vi "SP_Action_Taken_Report.vi"() -> ()   [LabVIEW 2017]
uses:
  <vilib>/addons/database/Connection.llb/DB Tools Open Connec (Path).vi
  Globle/Login Data.vi
  <vilib>/addons/database/NI_Database_API.lvlib
panel:
  in  "Cancel Button - Archive":bool
  out "Role Id":string
  out "stackholder":string
  in  "Download 2":bool
  in  "Get Rport":bool
  out "index of element":i32
  out "Table 2":string[][](array[string])
  in  "Station":string(combo)
  out "error out":errorcluster
  in  "error in (no error)":errorcluster
  out "Table":string[][](table)
  out "Run-Time Status":cluster{"Array 2":timestamp[], dbl[]}(graph)
  in  "Shift":string(combo)
  in  "To Date":timestamp format="%<%Y-%m-%d>T"
  in  "From Date":timestamp format="%<%Y-%m-%d>T"
  in  "Stakeholder":string(combo)
  # "Breakdown & Action Taken Report"
  # "Powered By - Infinity Automation Systems Pvt. Ltd."
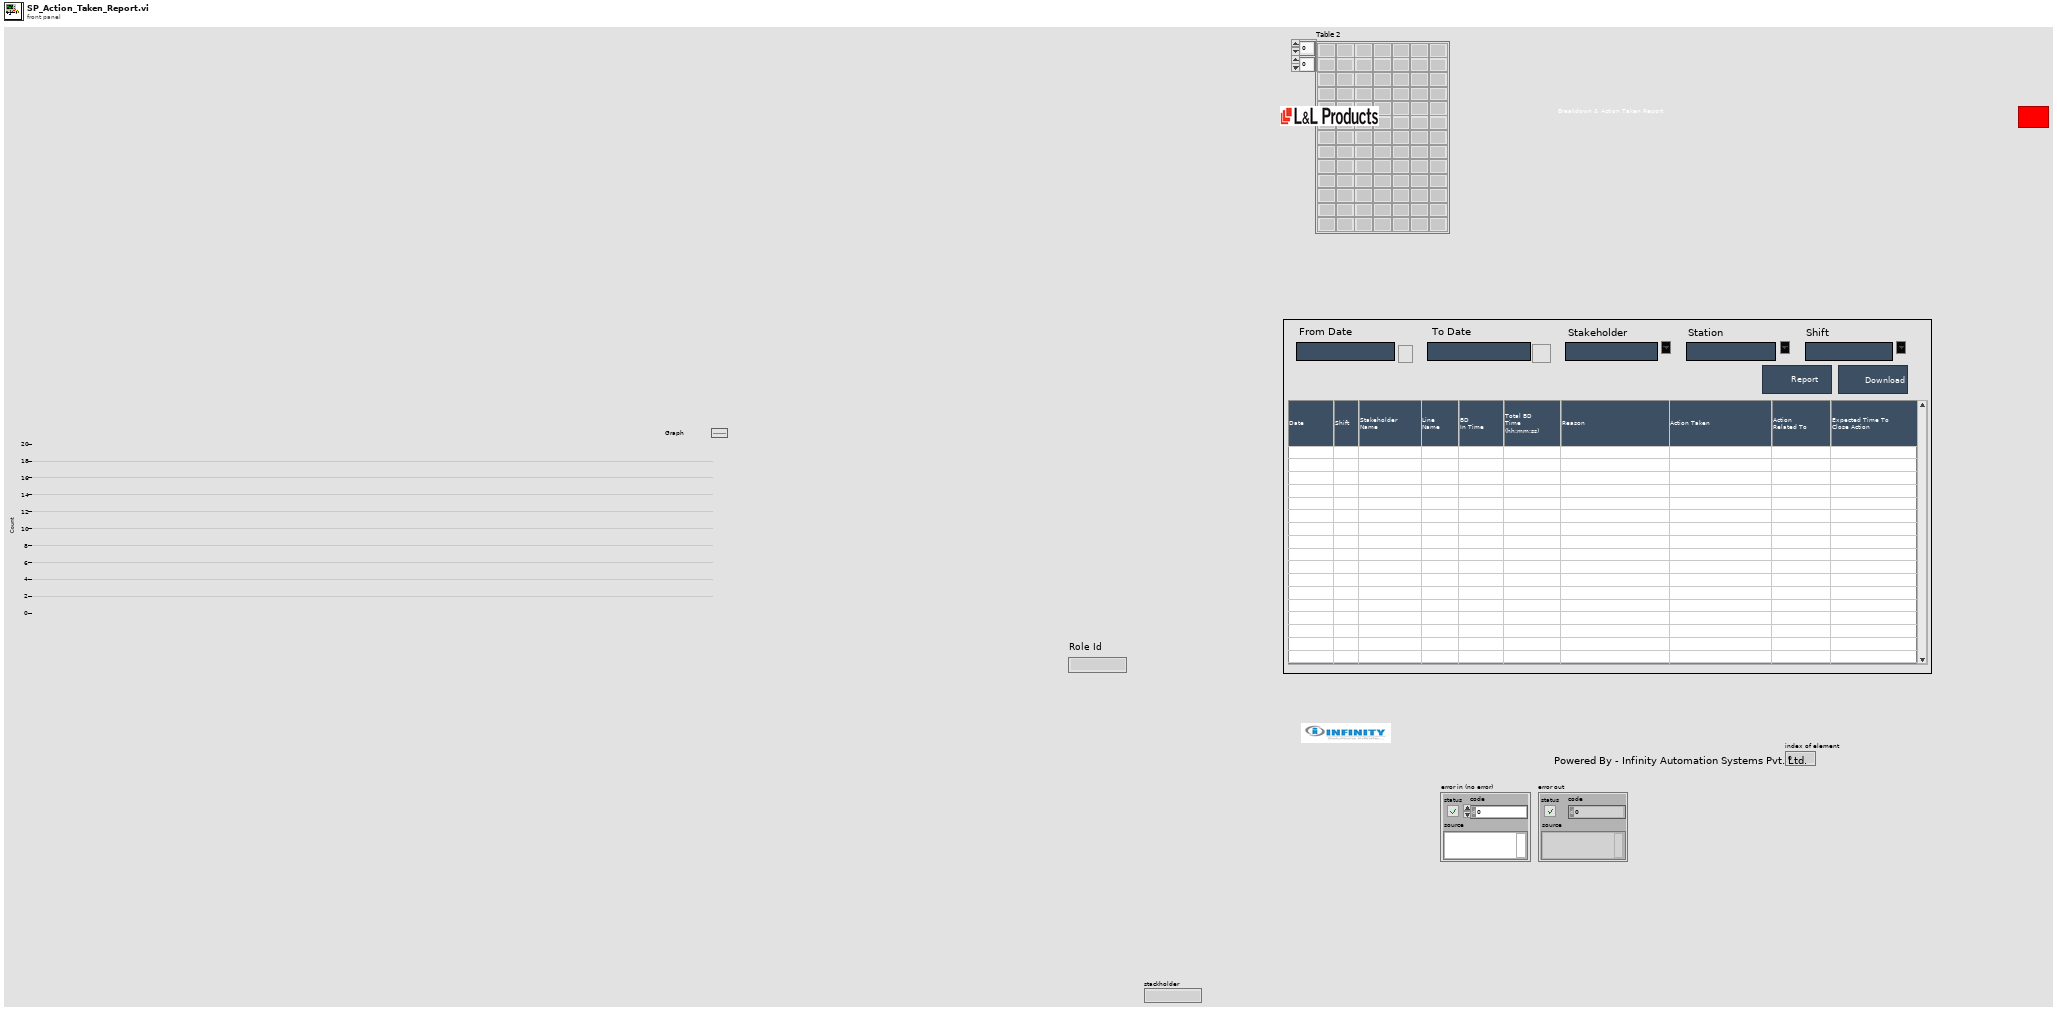
[diagram p1: front panel]
types:
  T1 = typedef "NI_Database_API.lvlib/Conn ObjectReference.ctl" = refnum<k1>
  T2 = enum32{"invalid app kind", "Development System", "Run Time System", "Student Edition", "Embedded LabVIEW", "Evaluation", "Custom"}
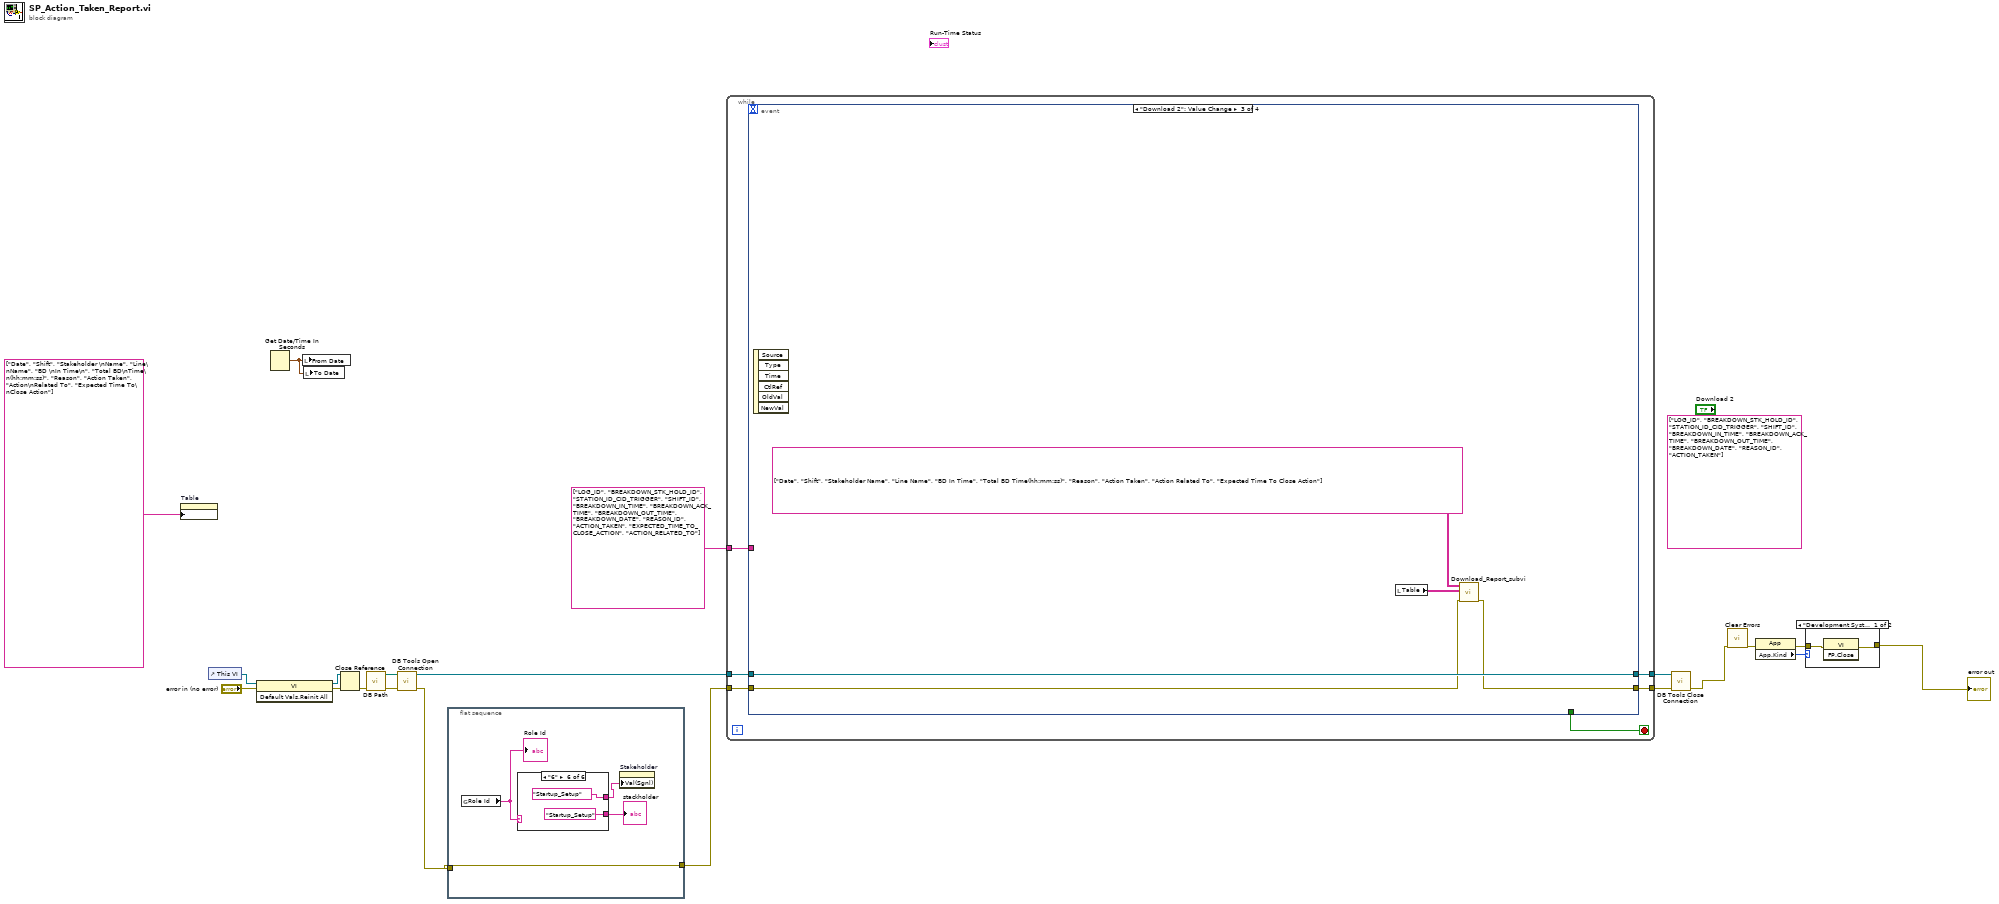
[diagram p0: block diagram]
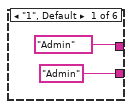
[diagram p2: hidden frame]
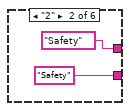
[diagram p3: hidden frame]
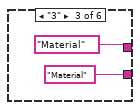
[diagram p4: hidden frame]
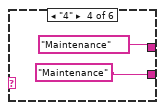
[diagram p5: hidden frame]
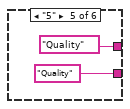
[diagram p6: hidden frame]
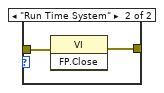
[diagram p7: hidden frame]
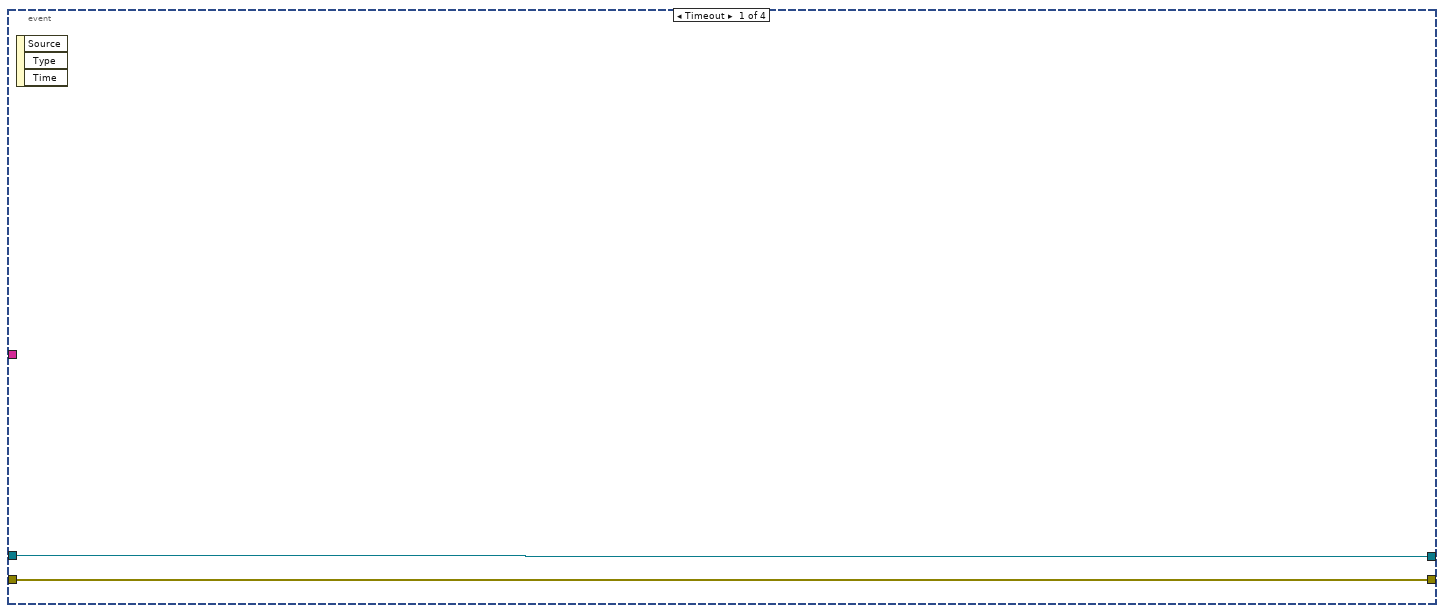
[diagram p8: hidden frame]
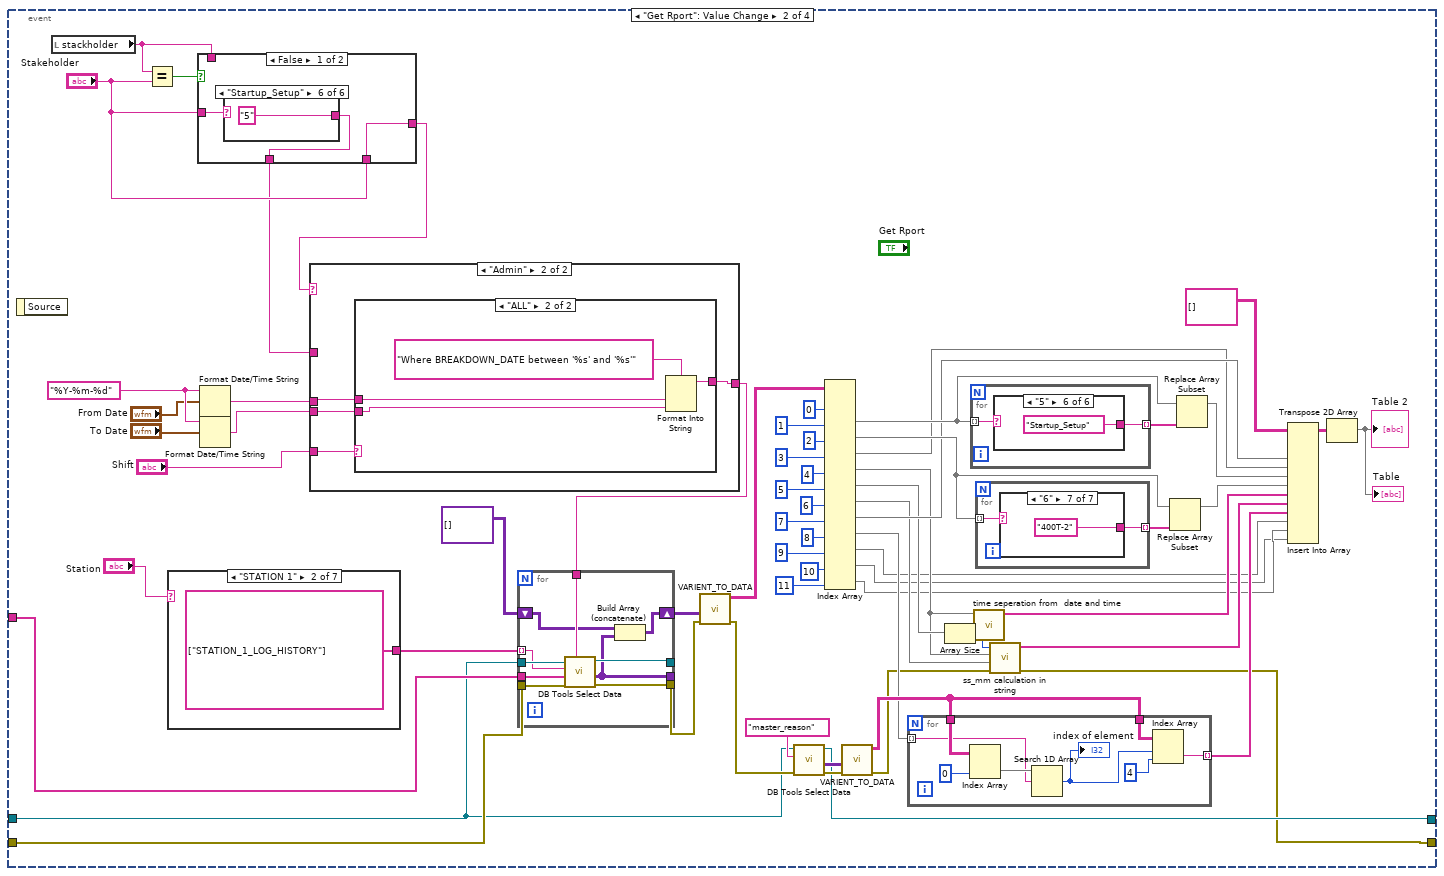
[diagram p9: hidden frame]
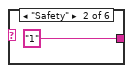
[diagram p11: hidden frame]
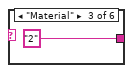
[diagram p12: hidden frame]
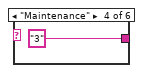
[diagram p13: hidden frame]
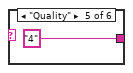
[diagram p14: hidden frame]
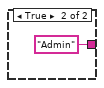
[diagram p15: hidden frame]
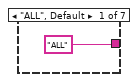
[diagram p16: hidden frame]
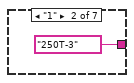
[diagram p17: hidden frame]
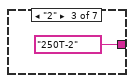
[diagram p18: hidden frame]
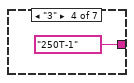
[diagram p19: hidden frame]
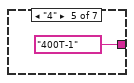
[diagram p20: hidden frame]
diagram:
  (unwired) string[] ["LOG_ID", "BREAKDOWN_STK_HOLD_ID", "STATION_ID_CID_TRIGGER", "SHIFT_ID", "BREAKDOWN_IN_TIME", "BREAKDOWN_ACK_TIME", "BREAKDOWN_OUT_TIME", "BREAKDOWN_DATE", "REASON_ID", "ACTION_TAKEN"]
  n1 = property on="Table" class="Tbl (strict)"("Column Headers[]"=string[] ["Date", "Shift", "Stakeholder \nName", "Line\nName", "BD \nIn Time\n", "Total BD\nTime\n(hh:mm:ss)", "Reason", "Action Taken", "Action\nRelated To", "Expected Time To\nClose Action"] ("Column Header Strings[]")) -> ()  [unwired: 2 in, 2 out]
  n2 = control-ref of="This VI"() -> (w20:refnum<vi>)
  n3 = invoke class="VI" method="Default Vals.Reinit All"(reference=w20, error in="error in (no error)") -> (reference out=w18:refnum<vi>, error out=w19:errorcluster)  [unwired: 1 in, 1 out]
  n4 = Get Date/Time In Seconds() -> (seconds since 1Jan1904=w9:timestamp)
  n5 = local write "From Date"(w9) -> ()
  n6 = local write "To Date"(w9) -> ()
  n7 = Close Reference(reference=w18, error in (no error)=w19) -> (error out=w17:errorcluster)
  n8 = call "DB Path.vi"("error in"=w17) -> ("error out"=w16:errorcluster, "DB Path"=w15:path)  [unwired: 9 in]
  n9 = call-poly <vilib>:"DB Tools Open Connection.vi"("error in (no error)"=w16, "connection information"=w15) -> ("error out"=w2:errorcluster, "connection reference"=w13:T1)  [unwired: 6 in]
  n10 = flat-sequence {
    tunnel: [w24] -> w1
    tunnel: w2 -> [w24]
    frame #0 {
      n11 = global read "Login Data.vi" "Role Id"() -> (w21:string)
      "Role Id" <- w21
      n12 = case shown="\"6\"" w21 {
        tunnel: ["Admin" ("string") "Safety" "Material" "Maintenance" "Quality" "Startup_Setup"] -> w22
        tunnel: ["Admin" ("Stakeholder") "Safety" ("Stakeholder") "Material" ("Stakeholder") "Maintenance" ("Stakeholder") "Quality" ("Stakeholder") "Startup_Setup" ("Stakeholder")] -> w23
        frame "1", Default {
        }
        frame "2" {
        }
        frame "3" {
        }
        frame "4" {
        }
        frame "5" {
        }
        frame "6" {
        }
      }
      "stackholder" <- w22
      n13 = property on="Stakeholder" class="CmbBox"("Val(Sgnl)"=w23) -> ()  [unwired: 2 in, 2 out]
    }
  }
  n14 = while {
    tunnel: w1 -> [w42]
    tunnel: [w41] -> w11
    tunnel: [w40] -> w10
    tunnel: w13 -> [w39]
    tunnel: string[] ["LOG_ID", "BREAKDOWN_STK_HOLD_ID", "STATION_ID_CID_TRIGGER", "SHIFT_ID", "BREAKDOWN_IN_TIME", "BREAKDOWN_ACK_TIME", "BREAKDOWN_OUT_TIME", "BREAKDOWN_DATE", "REASON_ID", "ACTION_TAKEN", "EXPECTED_TIME_TO_CLOSE_ACTION", "ACTION_RELATED_TO"] -> [w38]
    stop <- w37 stop-if-true
    n15 = event shown="[2] \"Download 2\": Value Change" {
      selector: _ -> [_ _ _ _]
      dyn-events: _ -> [_ _ _ _]
      timeout: _ -> [_ _ _ _]
      tunnel: [w44 w57 w189 w195] -> w41
      tunnel: w42 -> [w44 w98 w190 w195]
      tunnel: [w43 w60 w192 w194] -> w40
      tunnel: w39 -> [w43 w61 w192 w194]
      tunnel: w38 -> [_ w96 _ _]
      tunnel: [_ _ _ "Cancel Button - Archive"] -> w37
      event Timeout {
        n16 = event-data() -> ()  [unwired: 1 in, 3 out]
      }
      event "Get Rport": Value Change {
        w107 = "%Y-%m-%d" ("time format string (%c)")
        n17 = event-data() -> ()  [unwired: 1 in, 1 out]
        n18 = local read "stackholder"() -> (w49:string)
        n19 = Equal?(x=w49, y="Stakeholder") -> (x = y?=w53:bool)
        n20 = case shown="\"STATION 1\"" "Station" {
          tunnel: [string[] ["STATION_1_LOG_HISTORY", "STATION_2_LOG_HISTORY", "STATION_3_LOG_HISTORY", "STATION_4_LOG_HISTORY", "STATION_5_LOG_HISTORY", "STATION_6_LOG_HISTORY"] string[] ["STATION_1_LOG_HISTORY"] string[] ["STATION_2_LOG_HISTORY"] string[] ["STATION_3_LOG_HISTORY"] string[] ["STATION_4_LOG_HISTORY"] string[] ["STATION_5_LOG_HISTORY"] string[] ["STATION_6_LOG_HISTORY"]] -> w97
          frame "ALL", Default {
          }
          frame "STATION 1" {
          }
          frame "STATION 2" {
          }
          frame "STATION 3" {
          }
          frame "STATION 4" {
          }
          frame "STATION 5" {
          }
          frame "STATION 6" {
          }
        }
        n21 = case shown="False" w53 {
          tunnel: [w109 "Admin" ("Stakeholder")] -> w51
          tunnel: "Stakeholder" -> [w110 _]
          tunnel: w49 -> [_ _]
          tunnel: "Stakeholder" -> [w109 _]
          tunnel: [w108 _] -> w50
          frame False {
            n22 = case shown="\"Startup_Setup\"" w110 {
              tunnel: [_ "1" "2" "3" "4" "5"] -> w108
              frame "Admin", Default {
              }
              frame "Safety" {
              }
              frame "Material" {
              }
              frame "Maintenance" {
              }
              frame "Quality" {
              }
              frame "Startup_Setup" {
              }
            }
          }
          frame True {
          }
        }
        n23 = Format Date/Time String(time format string (%c)=w107, seconds (now)="From Date") -> (date/time string=w103:string)  [unwired: 1 in]
        n24 = Format Date/Time String(time format string (%c)=w107, seconds (now)="To Date") -> (date/time string=w102:string)  [unwired: 1 in]
        n25 = case shown="\"Admin\"" w51 {
          tunnel: [w162 w178] -> w99
          tunnel: "Shift" -> [w163 w177]
          tunnel: w103 -> [w161 w176]
          tunnel: w102 -> [w160 w175]
          tunnel: w50 -> [w159 _]
          frame "False", Default {
            n26 = case shown="\"ALL\"" w163 {
              selector: w163 -> [w164 _]
              tunnel: [w168 w173] -> w162
              tunnel: w161 -> [w167 w172]
              tunnel: w160 -> [w166 w171]
              tunnel: w159 -> [w165 w170]
              frame "False", Default {
                n27 = Format Into String(format string="Where BREAKDOWN_DATE between '%s' and '%s' and BREAKDOWN_STK_HOLD_ID ='%s'  and SHIFT_ID='%s'  " ("condition"), w167, w166, w165, w164) -> (resulting string=w168:string)  [unwired: 2 in, 1 out]
              }
              frame "ALL" {
                n28 = Format Into String(format string="Where BREAKDOWN_DATE between '%s' and '%s' and BREAKDOWN_STK_HOLD_ID = '%s' " ("condition"), w172, w171, w170) -> (resulting string=w173:string)  [unwired: 2 in, 1 out]
              }
            }
          }
          frame "Admin" {
            n29 = case shown="\"ALL\"" w177 {
              selector: w177 -> [w179 _]
              tunnel: [w182 w186] -> w178
              tunnel: w176 -> [w181 w185]
              tunnel: w175 -> [w180 w184]
              frame "False", Default {
                n30 = Format Into String(format string="Where BREAKDOWN_DATE between '%s' and '%s' and SHIFT_ID='%s'  " ("condition"), w181, w180, w179) -> (resulting string=w182:string)  [unwired: 2 in, 1 out]
              }
              frame "ALL" {
                n31 = Format Into String(format string="Where BREAKDOWN_DATE between '%s' and '%s'" ("condition"), w185, w184) -> (resulting string=w186:string)  [unwired: 2 in, 1 out]
              }
            }
          }
        }
        n32 = for {
          tunnel: w97 -> [w149] mode=indexing
          tunnel: [w143] -> _
          tunnel: w96 -> [w145]
          tunnel: w99 -> [w146]
          tunnel: w98 -> [w148]
          tunnel: [w147] -> w81
          tunnel: w61 -> [w151]
          tunnel: [w150] -> _
          shift-right: [w142] -> w80
          shift-left: variant[][] [] ("data") -> [w144]
          n33 = call <vilib>:"DB Tools Select Data.vi"("condition"=w146, "error in (no error)"=w148, "columns"=w145, "table"=w149, "connection reference"=w151) -> ("error out"=w147:errorcluster, "data"=w143:variant[][], "connection reference out"=w150:T1)  [unwired: 1 in]
          n34 = Build Array (concatenate)(w144, w143) -> (w142:variant[][])
        }
        n35 = call "VARIENT_TO_DATA.vi"("data"=w80, "error in (no error)"=w81) -> ("Table"=w79:string[][], "error out"=w65:errorcluster)  [unwired: 7 in]
        n36 = call <vilib>:"DB Tools Select Data.vi"("error in (no error)"=w65, "table"="master_reason", "connection reference"=w61) -> ("error out"=w67:errorcluster, "data"=w66:variant[][], "connection reference out"=w60:T1)  [unwired: 3 in]
        n37 = Index Array(array=w79, index (col) #1=0 ("disabled index (col)"), index (col) #2=1 ("disabled index (col)"), index (col) #3=2 ("disabled index (col)"), index (col) #4=3 ("disabled index (col)"), index (col) #5=4 ("disabled index (col)"), index (col) #6=5 ("disabled index (col)"), index (col) #7=6 ("disabled index (col)"), index (col) #8=7 ("disabled index (col)"), index (col) #9=8 ("disabled index (col)"), index (col) #10=9 ("disabled index (col)"), index (col) #11=10 ("disabled index (col)"), index (col) #12=11 ("disabled index (col)")) -> (element #2=w92:string[], element #3=w90:string[], element #4=w77:string[], element #5=w70:string[], element #6=w71:string[], element #7=w73:string[], element #8=w78:string[], element #9=w63:string[], element #10=w54:string[], element #11=w45:string[], element #12=w46:string[])  [unwired: 12 in, 1 out]
        n38 = call "VARIENT_TO_DATA.vi"("data"=w66, "error in (no error)"=w67) -> ("Table"=w64:string[][], "error out"=w58:errorcluster)  [unwired: 7 in]
        n39 = for {
          tunnel: [w120] -> w62 mode=indexing
          tunnel: w64 -> [w119]
          tunnel: w64 -> [w118]
          tunnel: w63 -> [w117] mode=indexing
          n40 = Index Array(array=w119, index (col)=0 ("disabled index (col)")) -> (element=w123:string[])  [unwired: 1 in]
          n41 = Search 1D Array(1D array=w123, element=w117) -> (index of element=w124:i32)  [unwired: 1 in]
          "index of element" <- w124
          n42 = Index Array(array=w118, index (row)=w124, index (col)=4 ("disabled index (col)")) -> (element=w120:string)
        }
        n43 = Array Size(array=w71) -> (size(s)=w72:i32)
        n44 = for {
          tunnel: w92 -> [w134] mode=indexing
          tunnel: [w135] -> w93 mode=indexing
          n45 = case shown="\"5\"" w134 {
            tunnel: ["all" "Safety" "Material" "Maintenance" "Quality" "Startup_Setup"] -> w135
            frame "False", Default {
            }
            frame "1" {
            }
            frame "2" {
            }
            frame "3" {
            }
            frame "4" {
            }
            frame "5" {
            }
          }
        }
        n46 = call "time seperation from  date and time.vi"("time and date"=w70) -> ("time array"=w74:string[])  [unwired: 10 in]
        n47 = for {
          tunnel: w90 -> [w125] mode=indexing
          tunnel: [w126] -> w89 mode=indexing
          n48 = case shown="\"6\"" w125 {
            tunnel: ["ALL" "250T-3" "250T-2" "250T-1" "400T-1" "150T-1" "400T-2"] -> w126
            frame "ALL", Default {
            }
            frame "1" {
            }
            frame "2" {
            }
            frame "3" {
            }
            frame "4" {
            }
            frame "5" {
            }
            frame "6" {
            }
          }
        }
        n49 = call "ss_mm calculation in string.vi"("error in (no error)"=w58, "Table 2"=w73, "Table"=w70, "Numeric"=w72) -> ("error out"=w57:errorcluster, "Array 2"=w69:string[])  [unwired: 6 in]
        n50 = Replace Array Subset(array=w90, new element=w89) -> (w75:string[])  [unwired: 1 in]
        n51 = Replace Array Subset(array=w92, new element=w93) -> (w76:string[])  [unwired: 1 in]
        n52 = Insert Into Array(array=string[][] [], new element #1=w78, new element #2=w77, new element #3=w76, new element #4=w75, new element #5=w74, new element #6=w69, new element #7=w62, new element #8=w54, new element #9=w46, new element #10=w45) -> (w83:string[][])  [unwired: 2 in]
        n53 = Transpose 2D Array(2D array=w83) -> (transposed array=→"Table 2" →"Table":string[][])
      }
      event "Download 2": Value Change {
        n54 = event-data() -> ()  [unwired: 1 in, 6 out]
        n55 = local read "Table"() -> (w188:string[][])
        n56 = call "Download_Report_subvi.vi"("error in (no error)"=w190, "Value"=w188, "Column Header Strings[]"=string[][] [["Date", "Shift", "Stakeholder Name", "Line Name", "BD In Time", "Total BD Time(hh:mm:ss)", "Reason", "Action Taken", "Action Related To", "Expected Time To Close Action"]]) -> ("error out"=w189:errorcluster)  [unwired: 8 in]
      }
      event "Cancel Button - Archive": Value Change {
        n57 = event-data() -> ()  [unwired: 1 in, 6 out]
      }
    }
  }
  n58 = call <vilib>:"DB Tools Close Connection.vi"("error in (no error)"=w11, "connection reference"=w10) -> ("error out"=w4:errorcluster)  [unwired: 5 in]
  n59 = call <vilib>:"Clear Errors.vi"("error in (no error)"=w4) -> ("error out"=w7:errorcluster)  [unwired: 5 in, 1 out]
  n60 = property class="App"(error in=w7) -> (error out=w6:errorcluster, "App.Kind"=w5:T2)  [unwired: 1 in, 1 out]
  n61 = case shown="\"Development System\", Default" w5 {
    tunnel: w6 -> [w197 w199]
    tunnel: [w196 w198] -> w3
    frame "Development System", Default {
      n62 = invoke class="VI" method="FP.Close"(error in=w197) -> (error out=w196:errorcluster)  [unwired: 2 in, 2 out]
    }
    frame "Run Time System" {
      n63 = invoke class="VI" method="FP.Close"(error in=w199) -> (error out=w198:errorcluster)  [unwired: 2 in, 2 out]
    }
  }
  "error out" <- w3
